vi "Alphs Blend Glyphs __jki_lib_picture -- VI Tester.vi"(7 "error in (no error)":errorcluster, 8 "Background color (White)":u32(colorbox)=16777215, 9 "Transparency Thresh (127)":u8=127, 10 "image data in":T1) -> (0 "error out":errorcluster, 3 "image data out":T1)   [LabVIEW 2011]
uses:
  <vilib>/picture/picture.llb/imagedata.ctl
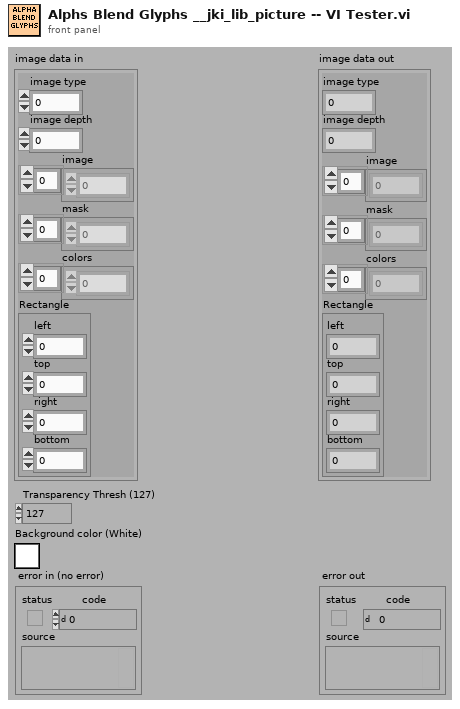
[diagram p1: front panel]
types:
  T1 = typedef "imagedata.ctl" = cluster{"image type":i32, "image depth":i32, "image":u8[], "mask":u8[], "colors":u32[], "Rectangle":cluster{"left":i16, "top":i16, "right":i16, "bottom":i16}}
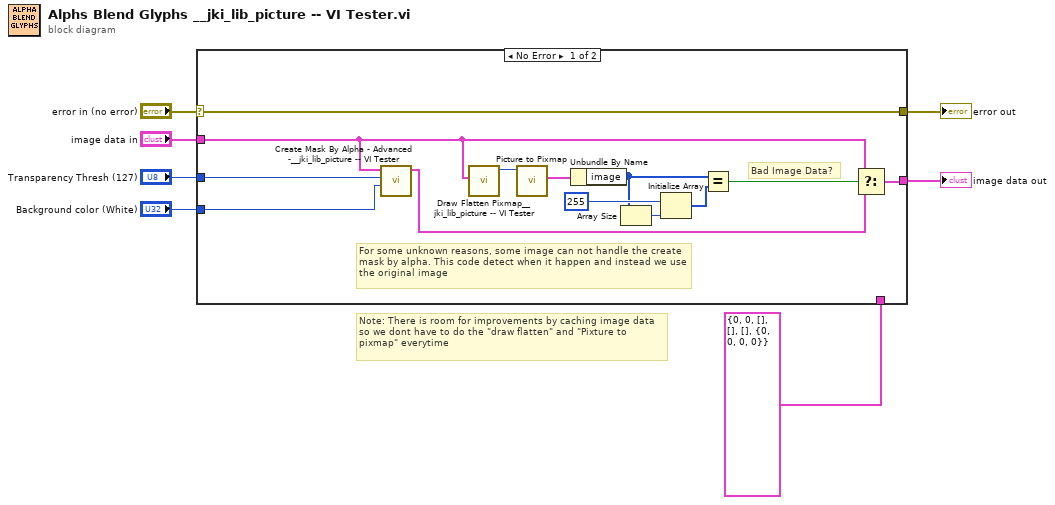
[diagram p0: block diagram]
diagram:
  # "Note: There is room for improvements by caching image data so we dont have to do the \"draw flatten\" and \"Pixture to pixmap\" everytime"
  n1 = case shown="No Error" "error in (no error)" {
    selector: "error in (no error)" -> [w9 w22]
    tunnel: "image data in" -> [w10 _]
    tunnel: [w20 w21] -> w3
    tunnel: [w9 w22] -> w6
    tunnel: T1 {"image type"=0, "image depth"=0, "image"=[], "mask"=[], "colors"=[], "Rectangle"={"left"=0, "top"=0, "right"=0, "bottom"=0}} ("image data") -> [_ w21]
    tunnel: "Transparency Thresh (127)" -> [w19 _]
    tunnel: "Background color (White)" -> [w8 _]
    frame No Error {
      # "For some unknown reasons, some image can not handle the create mask by alpha. This code detect when it happen and instead we use the original image"
      # "Bad Image Data?"
      n2 = call "Create Mask By Alpha - Advanced -__jki_lib_picture -- VI Tester.vi"("Background color (White)"=w8, "Transparency Thresh"=w19, "image data"=w10) -> ("masked image data"=w11:T1)  [unwired: 8 in]
      n3 = call "Draw Flatten Pixmap__jki_lib_picture -- VI Tester.vi"("image data"=w10) -> ("new picture"=w13:picture)  [unwired: 10 in]
      n4 = call <vilib>:"Picture to Pixmap.vi"("picture"=w13) -> ("image data"=w12:T1)  [unwired: 9 in, 1 out]
      n5 = Unbundle By Name(w12) -> ("image"=w15:u8[])
      n6 = Array Size(array=w15) -> (size(s)=w18:i32)
      n7 = Initialize Array(u8 255, w18) -> (w16:u8[])
      n8 = Equal?(x=w15, y=w16) -> (x = y?=w14:bool)
      n9 = Select(t=w10, s=w14, f=w11) -> (s? t:f=w20:T1)
    }
    frame Error {
    }
  }
  "image data out" <- w3
  "error out" <- w6
